vi "Main.vi"   [LabVIEW 2017]
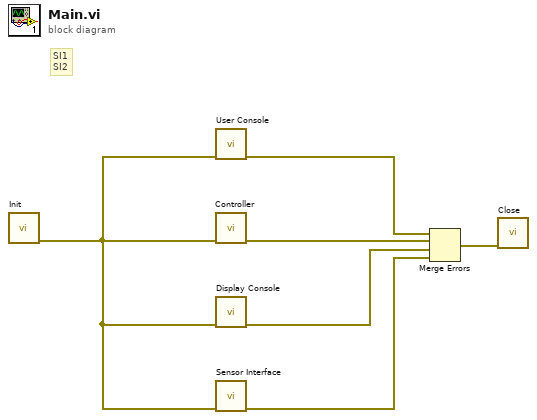
[diagram p0: block diagram]
diagram:
  # "SI1\nSI2"
  n1 = call "Init.vi"() -> ("error out"=w6:errorcluster)  [unwired: 11 in]
  n2 = call "User Console.vi"("error in (no error)"=w6) -> ("error out"=w5:errorcluster)  [unwired: 10 in]
  n3 = call "Controller.vi"("Error In"=w6) -> ("Error Out"=w4:errorcluster)  [unwired: 10 in]
  n4 = call "Display Console.vi"("Error In"=w6) -> ("Error Out"=w3:errorcluster)  [unwired: 10 in]
  n5 = call "Sensor Interface.vi"("Error In"=w6) -> ("Error Out"=w2:errorcluster)  [unwired: 10 in]
  n6 = Merge Errors(w5, w4, w3, w2) -> (w1:errorcluster)
  n7 = call "Close.vi"("error in (no error)"=w1) -> ()  [unwired: 10 in, 1 out]
